vi "MPExxx_get_modulation_table.vi"(0 "VISA session":refnum<visa-resource-name>, 1 "Row":i8=1 min=1 max=20 step=1, 2 "error in (no error)":errorcluster) -> (3 "dup VISA session":refnum<visa-resource-name>, 4 "Modulation Voltage":dbl format="%.3f", 5 "Modulation Factor":dbl format="%.3f", 6 "error out":errorcluster)   [LabVIEW 2012]
doc: "This VI form returns the modulation parameters (modulation voltage and modulation factor) for the specified row."
uses:
  MPExxx Globals.gbl
panel:
  # "MAGNA-POWER"
  # "Electronics"
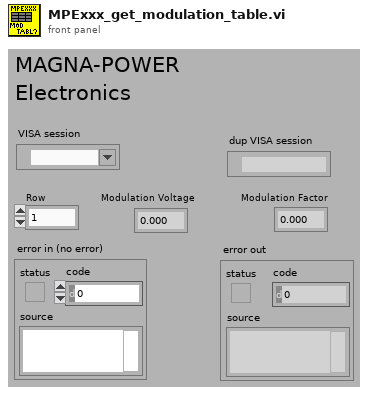
[diagram p1: front panel]
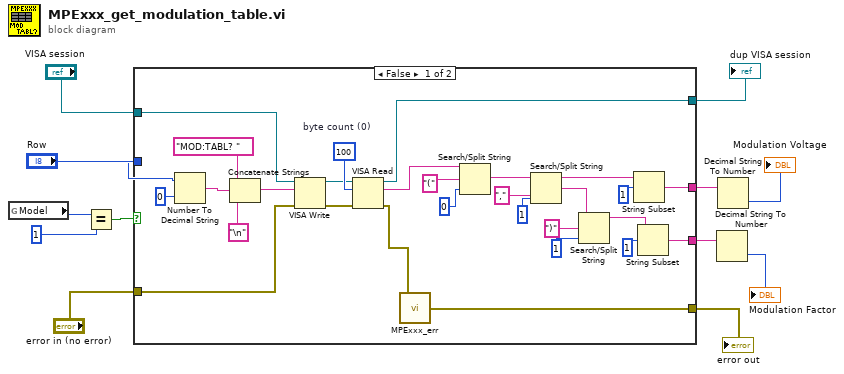
[diagram p0: block diagram]
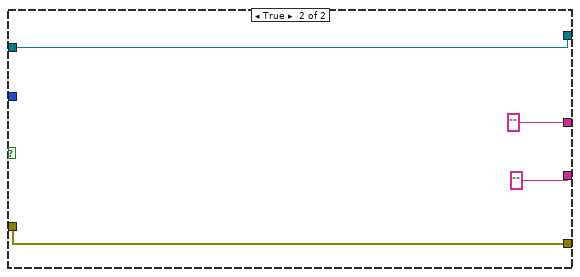
[diagram p2: hidden frame]
diagram:
  n1 = global read "MPExxx Globals.gbl" "Model"() -> (w10:u8)
  n2 = Equal?(x=w10, y=1) -> (x = y?=w12:bool)
  n3 = case shown="False" w12 {
    tunnel: "VISA session" -> [w20 w45]
    tunnel: "error in (no error)" -> [w19 w44]
    tunnel: [w18 w45] -> w7
    tunnel: [w17 w44] -> w6
    tunnel: [w16 ""] -> w3
    tunnel: [w15 ""] -> w4
    tunnel: "Row" -> [w14 _]
    frame False {
      w29 = u32 100  # byte count (0)
      n4 = Number To Decimal String(number=w14, width (-)=0) -> (decimal integer string=w23:string)
      n5 = Concatenate Strings("MOD:TABL? ", w23, "\n") -> (w21:string)
      n6 = VISA Write(VISA resource name=w20, write buffer=w21, error in (no error)=w19) -> (VISA resource name out=w27:refnum<visa-resource-name>, error out=w28:errorcluster)  [unwired: 1 out]
      n7 = VISA Read(VISA resource name=w27, byte count=w29, error in (no error)=w28) -> (VISA resource name out=w18:refnum<visa-resource-name>, read buffer=w13:string, error out=w26:errorcluster)  [unwired: 1 out]
      n8 = call "MPExxx_err.vi"("error in (no error)"=w26) -> ("error out"=w17:errorcluster)
      n9 = Search/Split String(string=w13, search string/char (-)="(", offset (0)=0) -> (match + rest of string=w35:string)  [unwired: 2 out]
      n10 = Search/Split String(string=w35, search string/char (-)=",", offset (0)=1) -> (substring before match=w33:string, match + rest of string=w34:string)  [unwired: 1 out]
      n11 = Search/Split String(string=w34, search string/char (-)=")", offset (0)=1) -> (substring before match=w30:string)  [unwired: 2 out]
      n12 = String Subset(string=w33, offset (0)=1) -> (substring=w15:string)  [unwired: 1 in]
      n13 = String Subset(string=w30, offset (0)=1) -> (substring=w16:string)  [unwired: 1 in]
    }
    frame True {
    }
  }
  "error out" <- w6
  "dup VISA session" <- w7
  n14 = Decimal String To Number(string=w3) -> (number=→"Modulation Factor":i32)  [unwired: 2 in, 1 out]
  n15 = Decimal String To Number(string=w4) -> (number=→"Modulation Voltage":i32)  [unwired: 2 in, 1 out]
